vi "Part 1.vi"(11 "Input":string) -> (3 "Output":i64)   [LabVIEW 2021]
uses:
  <userlib>/_OpenG.lib/string/string.llb/Convert EOLs (String)__ogtk.vi
  <vilib>/regexp/Match Regular Expression.xnode
panel:
  # "553825"
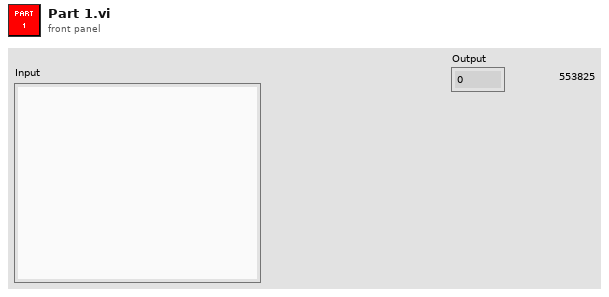
[diagram p1: front panel]
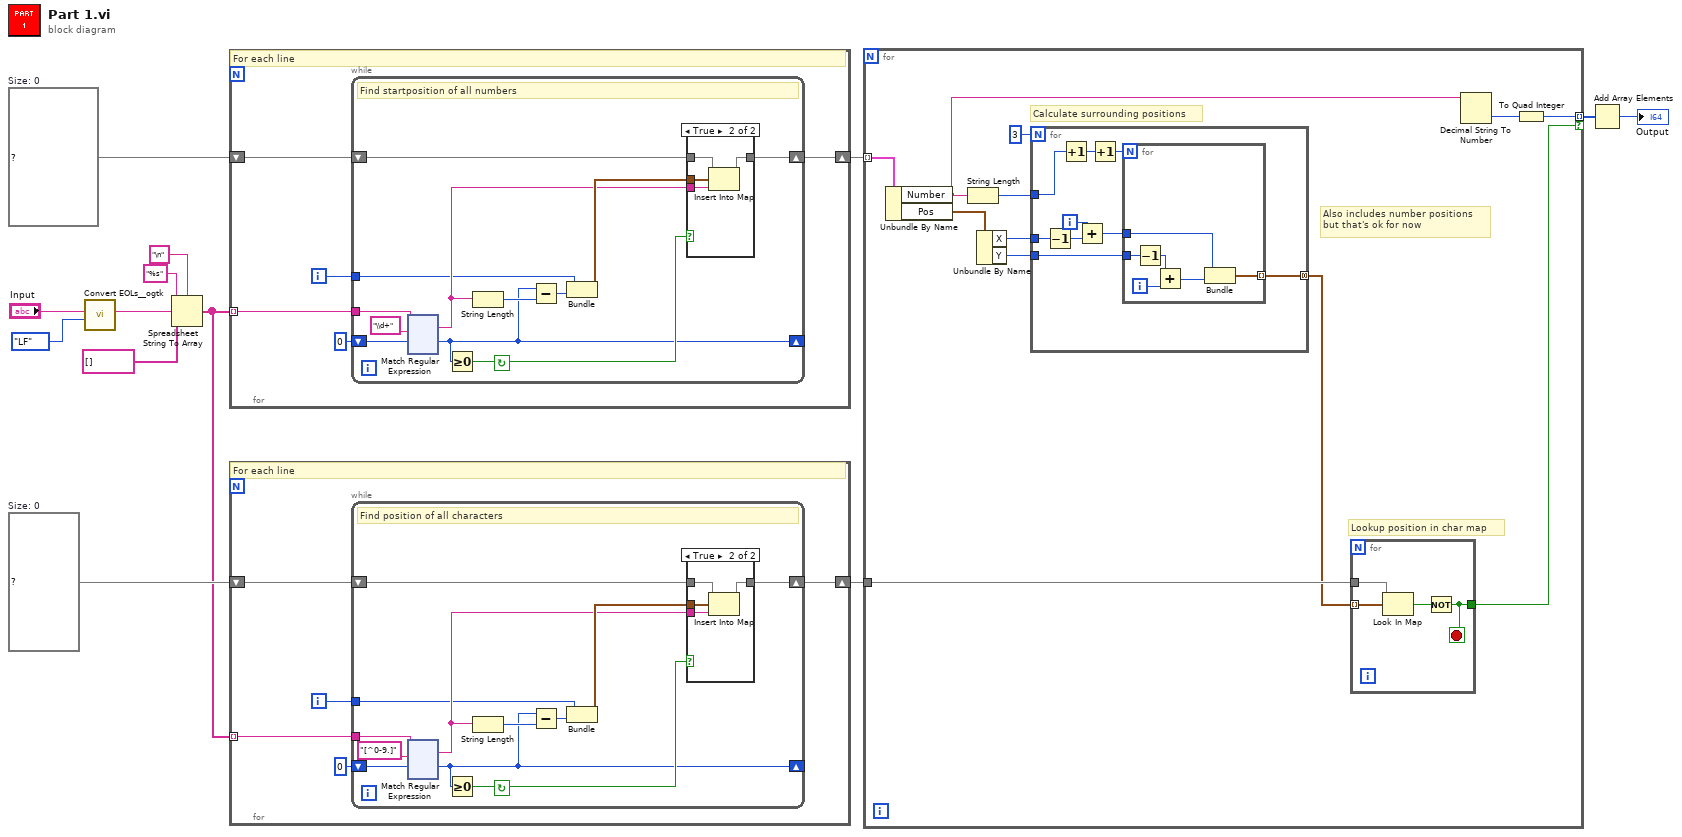
[diagram p0: block diagram]
diagram:
  w7 = map{cluster{"X":i32, "Y":i32}, string} {}  # Size: 0
  w3 = map{cluster{"X":i32, "Y":i32}, string} {}  # Size: 0
  n1 = call-poly <userlib>:"Convert EOLs__ogtk.vi"("Convert to:"=enum16{"CR", "LF", "CRLF"}."LF", "String in"="Input") -> ("String out"=w9:string)  [unwired: 9 in]
  n2 = Spreadsheet String To Array(delimiter (Tab)="\n", format string="%s", spreadsheet string=w9, array type (2D Dbl)=string[] []) -> (array=w2:string[])
  n3 = for {
    tunnel: w2 -> [w18] mode=indexing
    shift-right: [w14] -> w6
    shift-left: w7 -> [w15]
    i -> [w16]
    # "For each line"
    n4 = while {
      tunnel: w18 -> [w28]
      shift-right: [w20] -> _
      shift-left: 0 -> [w27]
      tunnel: w16 -> [w21]
      shift-right: [w25] -> w14
      shift-left: w15 -> [w26]
      stop <- w23 continue-if-true
      # "Find startposition of all numbers"
      n5 = xnode "Match Regular Expression"("input string"=w28, "regular expression"="\\d+", "offset (0)"=w27) -> ("whole match"=w22:string, "offset past match"=w20:i32)  [unwired: 3 in, 3 out]
      n6 = Greater Or Equal To 0?(x=w20) -> (x >= 0?=w23:bool)
      n7 = String Length(string=w22) -> (length=w30:i32)
      n8 = Subtract(x=w20, y=w30) -> (x-y=w29:i32)
      n9 = Bundle(w21, w29) -> (w24:cluster{i32, i32})  [unwired: 1 in]
      n10 = case shown="True" w23 {
        tunnel: w24 -> [_ w35]
        tunnel: w26 -> [w31 w34]
        tunnel: [w31 w33] -> w25
        tunnel: w22 -> [_ w32]
        frame False {
        }
        frame True {
          n11 = Insert Into Map(map in=w34, key=w35, value=w32) -> (map out=w33:map{cluster{"X":i32, "Y":i32}, string})  [unwired: 2 out]
        }
      }
    }
  }
  n12 = for {
    tunnel: w2 -> [w157] mode=indexing
    shift-right: [w153] -> w1
    shift-left: w3 -> [w154]
    i -> [w155]
    # "For each line"
    n13 = while {
      tunnel: w157 -> [w167]
      shift-right: [w159] -> _
      shift-left: 0 -> [w166]
      tunnel: w155 -> [w160]
      shift-right: [w164] -> w153
      shift-left: w154 -> [w165]
      stop <- w162 continue-if-true
      # "Find position of all characters"
      n14 = xnode "Match Regular Expression"("input string"=w167, "regular expression"="[^0-9.]", "offset (0)"=w166) -> ("whole match"=w161:string, "offset past match"=w159:i32)  [unwired: 3 in, 3 out]
      n15 = Greater Or Equal To 0?(x=w159) -> (x >= 0?=w162:bool)
      n16 = String Length(string=w161) -> (length=w169:i32)
      n17 = Subtract(x=w159, y=w169) -> (x-y=w168:i32)
      n18 = Bundle(w160, w168) -> (w163:cluster{i32, i32})  [unwired: 1 in]
      n19 = case shown="True" w162 {
        tunnel: w163 -> [_ w174]
        tunnel: w165 -> [w170 w173]
        tunnel: [w170 w172] -> w164
        tunnel: w161 -> [_ w171]
        frame False {
        }
        frame True {
          n20 = Insert Into Map(map in=w173, key=w174, value=w171) -> (map out=w172:map{cluster{"X":i32, "Y":i32}, string})  [unwired: 2 out]
        }
      }
    }
  }
  n21 = for {
    tunnel: w6 -> [w303] mode=indexing
    tunnel: w1 -> [w297]
    tunnel: [w292] -> w5 mode=indexing if=w293
    # "Also includes number positions\nbut that's ok for now"
    # "Lookup position in char map"
    # "Calculate surrounding positions"
    n22 = Unbundle By Name(w303) -> ("Number"=w295:string, "Pos"=w301:cluster{"X":i32, "Y":i32})
    n23 = String Length(string=w295) -> (length=w298:i32)
    n24 = Unbundle By Name(w301) -> ("X"=w300:i32, "Y"=w299:i32)
    n25 = for {
      N: 3 -> [_]
      tunnel: w300 -> [w316]
      tunnel: w299 -> [w312]
      tunnel: w298 -> [w311]
      tunnel: [w308] -> w296 mode=concatenating
      i -> [w314]
      n26 = Decrement(x=w316) -> (x-1=w315:i32)
      n27 = Increment(x=w311) -> (x+1=w310:i32)
      n28 = Add(x=w314, y=w315) -> (x+y=w313:i32)
      n29 = Increment(x=w310) -> (x+1=w309:i32)
      n30 = for {
        N: w309 -> [_]
        tunnel: w313 -> [w318]
        tunnel: w312 -> [w322]
        tunnel: [w317] -> w308 mode=indexing
        i -> [w321]
        n31 = Decrement(x=w322) -> (x-1=w320:i32)
        n32 = Add(x=w320, y=w321) -> (x+y=w319:i32)
        n33 = Bundle(w318, w319) -> (w317:cluster{i32, i32})  [unwired: 1 in]
      }
    }
    n34 = for {
      tunnel: w297 -> [w307]
      tunnel: w296 -> [w306] mode=indexing
      tunnel: [w304] -> w293
      stop <- w304 stop-if-true
      n35 = Look In Map(map=w307, key=w306) -> (key not found?=w305:bool)  [unwired: 1 in, 1 out]
      n36 = Not(x=w305) -> (.not. x?=w304:bool)
    }
    n37 = Decimal String To Number(string=w295) -> (number=w294:i32)  [unwired: 2 in, 1 out]
    n38 = To Quad Integer(1:w294) -> (0:w292:i64)
  }
  n39 = Add Array Elements(numeric array=w5) -> (sum=→"Output":i64)
